vi "ClusterToArray.vi"(11 "Cluster":variant) -> (3 "Array":variant[](array[variant]))   [LabVIEW 2013]
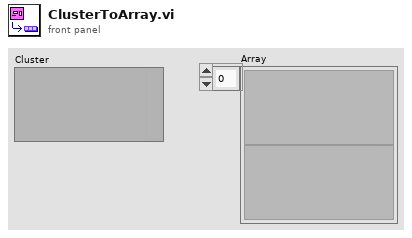
[diagram p1: front panel]
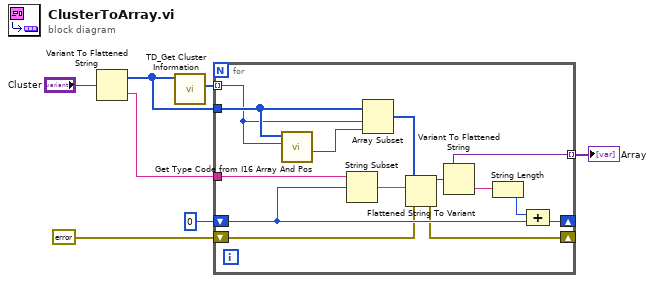
[diagram p0: block diagram]
diagram:
  n1 = Variant To Flattened String(Variant="Cluster") -> (data string=w5:string, 1:w3:i16[])
  n2 = call <vilib>:"TD_Get Cluster Information.vi"("Type descriptor"=w3) -> ("Contained TD Offsets"=w2:i32[])  [unwired: 9 in, 1 out]
  n3 = for {
    tunnel: w3 -> [w11]
    shift-right: [w15] -> _
    shift-left: 0 -> [w16]
    tunnel: w5 -> [w20]
    tunnel: [w14] -> w6 mode=indexing
    shift-right: [w12] -> _
    shift-left: errorcluster {"status"=FALSE, "code"=0, "source"=""} ("error out") -> [w13]
    tunnel: w2 -> [w9] mode=indexing
    n4 = call <vilib>:"Get Type Code from I16 Array And Pos.vi"("Pos in Type Descriptor (0)"=w9, "Type descriptor"=w11) -> ("Size (Words)"=w10:i32)  [unwired: 7 in, 2 out]
    n5 = String Subset(string=w20, offset (0)=w16) -> (substring=w19:string)  [unwired: 1 in]
    n6 = Array Subset(array=w11, index=w9, length=w10) -> (w8:i16[])
    n7 = Flattened String To Variant(4:w13, 6:w19, 7:w8) -> (0:w12:errorcluster, 3:w14:variant)
    n8 = Variant To Flattened String(Variant=w14) -> (data string=w18:string)  [unwired: 1 out]
    n9 = String Length(string=w18) -> (length=w17:i32)
    n10 = Compound Arithmetic op=ADD(w17, w16) -> (w15:i32)
  }
  "Array" <- w6
